vi "ProSCI Global.vi"() -> ()   [LabVIEW 2012]
panel:
  in  "gPreImagingDelay":i32
  in  "gForwardDelay":i32
  in  "gFLLampOffDelay":i32
  in  "gFLLampOnDelay":i32
  in  "gBFLampOffDelay":i32
  in  "gFLExpTime 6":dbl[](array[numeric])
  in  "gFLExpTime 5":dbl[](array[numeric])
  in  "gFLExpTime 4":dbl[](array[numeric])
  in  "gFLExpTime 3":dbl[](array[numeric])
  in  "gFLExpTime 2":dbl[](array[numeric])
  in  "gFLExcitationFilter":i8
  in  "gFLExcite6":bool
  in  "gFLExcite5":bool
  in  "gFLExcite4":bool
  in  "gFLExcite3":bool
  in  "gFLExcite2":bool
  in  "gFLExcite1":bool
  in  "gFLExpTime":dbl[](array[numeric])
  in  "gCurrentExpTime":dbl[](array[numeric])
  in  "gBFExpTime":dbl[](array[numeric])
  out "gMultiFluoExp":bool
  in  "gFluoExpArray":dbl[](array[numeric])
  out "gThumbThis":bool
  out "gAttachImage":bool
  in  "gNotify":enum16{"None", "Email", "SMS", "Both"}(ring)
  out "gNotifyEvery":u32
  out "gSMSID":string
  out "gEmailID":string
  out "gMag":u8
  out "gObj":u8
  out "gGlobalOffsetY":i32
  out "gGlobalOffsetX":i32
  out "gImageMono":bool
  out "gFileTileSuffix":string
  out "gLogFileRef":refnum<file>
  in  "gNextPass":u16(ring) items=["Brightfield", "Fluorescence", "Both"]
  in  "gThisPass":u16(ring) items=["Brightfield", "Fluorescence", "Both"]
  out "gLubRun":i32
  out "gKnifeRun":i32
  out "gEventLog":string[](array[string])
  in  "gAppsStopped":u8
  out "gSaveImages":bool
  in  "gStop All":bool
  out "gCutSequenceOn":bool
  out "gGrabbing":bool
  out "gQCamHeartbeat":u32
  in  "gBFLampOnDelay":i32
  in  "gCutsCompleted":i32
  in  "gBrLampIntensity":u8
  out "gFlLampOn":bool
  out "gBrLampOn":bool
  in  "gIntervalCounted":i32
  in  "gFlExpMem":dbl
  in  "gBrExpMem":dbl
  in  "gImageInterval":i32
  in  "gIntervalMode":i8
  in  "gImageType":i8
  out "gImageTaken":bool
  in  "gExpTimeSendToCamera":dbl
  in  "gFullFileName":string
  in  "gGrabImage":bool
  out "gBaseFile":string
  out "gBaseDir":string
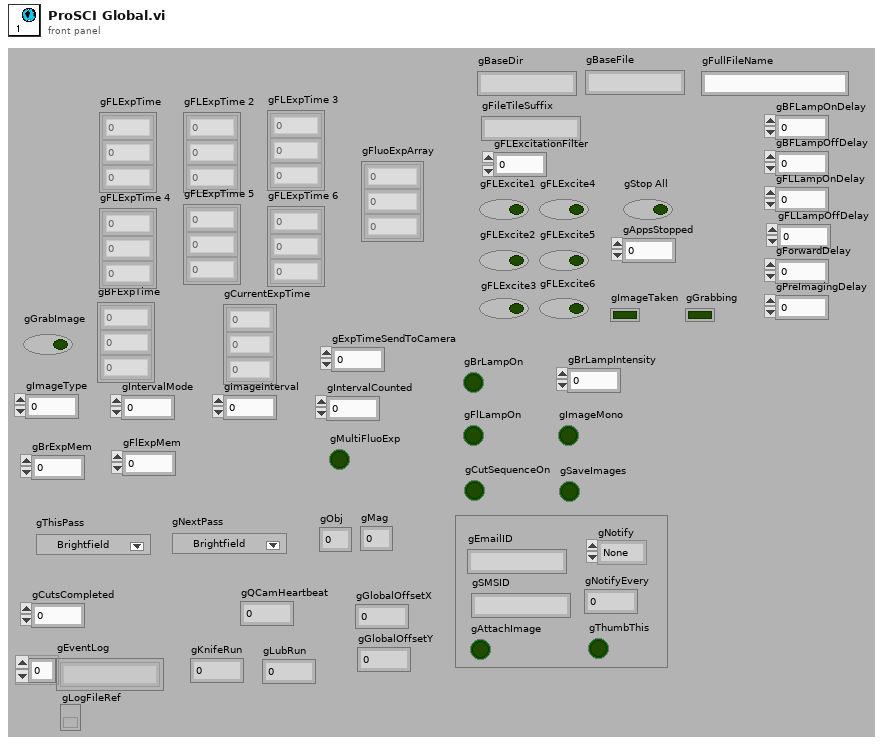
[diagram p1: front panel]
diagram:
